vi "Find Midpoint.vi"(8 "error in (no error)":errorcluster, 10 "Image In":T1, 11 "Gantry Class in":refnum<class "Gantry Class.lvclass">) -> (0 "error out":errorcluster, 1 "Vec3d Class out":refnum<class "Vec3d Class.lvclass">, 2 "Image Out":T1, 3 "Gantry Class out":refnum<class "Gantry Class.lvclass">)   [LabVIEW 2017, in "Gantry Class.lvclass"]
uses:
  Gantry Class.lvclass
  Vec3d Class/Vec3d Class.lvclass
  Config Manager Class/Type Definitions/Camera Enum.ctl
  <vilib>/vision/Image Controls.llb/IMAQ Image.ctl
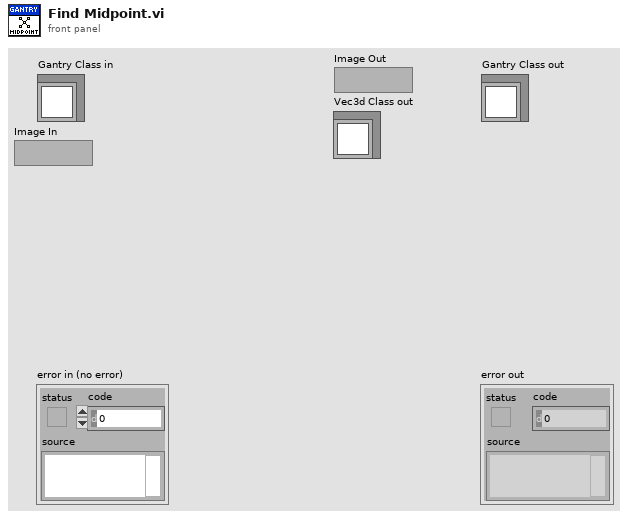
[diagram p1: front panel]
types:
  T1 = typedef "IMAQ Image.ctl" = refnum<image>
  T2 = typedef "Camera Enum.ctl" = enum16{"gantryhead", "NEEDLE CALIBRATION X", "NEEDLE CALIBRATION Y", "STAND CAMERA", "SIMRAN WEBCAM"}
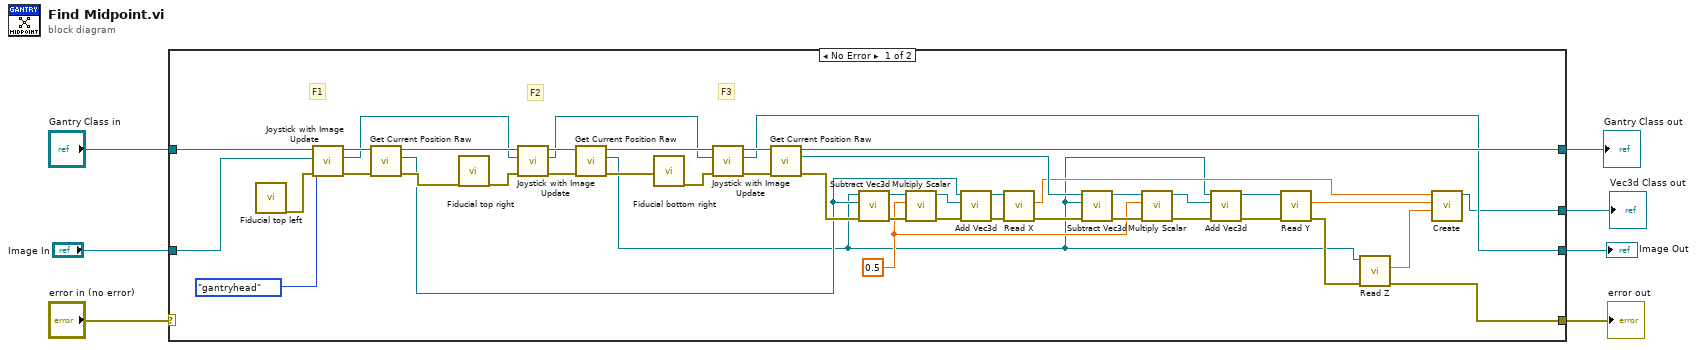
[diagram p0: block diagram]
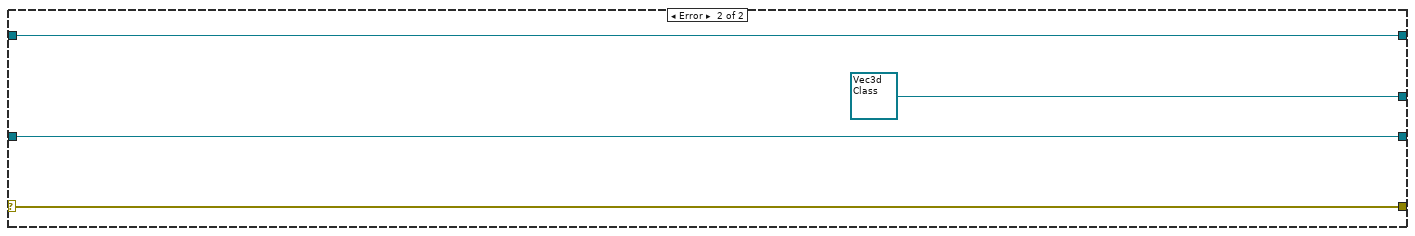
[diagram p2: hidden frame]
diagram:
  n1 = case shown="No Error" "error in (no error)" {
    selector: "error in (no error)" -> [_ w55]
    tunnel: [w24 w55] -> w6
    tunnel: "Gantry Class in" -> [w30 w54]
    tunnel: "Image In" -> [w29 w53]
    tunnel: [w26 w53] -> w3
    tunnel: [w27 w54] -> w2
    tunnel: [w20 refnum<class "Vec3d Class.lvclass"> refnum ("Vec3d Class out")] -> w1
    frame No Error {
      w12 = 0.5 ("Scale")
      # "F3"
      # "F2"
      # "F1"
      n2 = call "Fiducial top left"() -> ("error out"=w49:errorcluster)  [unwired: 18 in, 1 out]
      n3 = call-dynamic "Joystick with Image Update.vi"("error in (no error)"=w49, "Camera Name"=Camera_Enum."gantryhead", "Image In"=w29, "Gantry Class in"=w30) -> ("error out"=w50:errorcluster, "Image Out"=w32:T1, "Gantry Class out"=w51:refnum<class "Gantry Class.lvclass">)  [unwired: 5 in]
      n4 = call-dynamic "Get Current Position Raw.vi"("error in"=w50, "Gantry in"=w51) -> ("error out"=w44:errorcluster, "Vec3d Class out"=w10:refnum<class "Vec3d Class.lvclass">, "Gantry out"=w45:refnum<class "Gantry Class.lvclass">)  [unwired: 7 in]
      n5 = call "Fiducial top right"("error in (no error)"=w44) -> ("error out"=w46:errorcluster)  [unwired: 17 in, 1 out]
      n6 = call-dynamic "Joystick with Image Update.vi"("error in (no error)"=w46, "Image In"=w32, "Gantry Class in"=w45) -> ("error out"=w47:errorcluster, "Image Out"=w31:T1, "Gantry Class out"=w48:refnum<class "Gantry Class.lvclass">)  [unwired: 6 in]
      n7 = call-dynamic "Get Current Position Raw.vi"("error in"=w47, "Gantry in"=w48) -> ("error out"=w40:errorcluster, "Vec3d Class out"=w8:refnum<class "Vec3d Class.lvclass">, "Gantry out"=w39:refnum<class "Gantry Class.lvclass">)  [unwired: 7 in]
      n8 = call "Fiducial bottom right"("error in (no error)"=w40) -> ("error out"=w41:errorcluster)  [unwired: 17 in, 1 out]
      n9 = call-dynamic "Joystick with Image Update.vi"("error in (no error)"=w41, "Image In"=w31, "Gantry Class in"=w39) -> ("error out"=w42:errorcluster, "Image Out"=w26:T1, "Gantry Class out"=w43:refnum<class "Gantry Class.lvclass">)  [unwired: 6 in]
      n10 = call-dynamic "Get Current Position Raw.vi"("error in"=w42, "Gantry in"=w43) -> ("error out"=w34:errorcluster, "Vec3d Class out"=w37:refnum<class "Vec3d Class.lvclass">, "Gantry out"=w27:refnum<class "Gantry Class.lvclass">)  [unwired: 7 in]
      n11 = call "Subtract Vec3d.vi"("error in (no error)"=w34, "Vec3d in 2"=w10, "Vec3d in 1"=w8) -> ("error out"=w36:errorcluster, "Vec3d Class out"=w19:refnum<class "Vec3d Class.lvclass">)  [unwired: 7 in]
      n12 = call-dynamic "Multiply Scalar.vi"("error in"=w36, "Scale"=w12, "Vec3d in"=w19) -> ("error out"=w18:errorcluster, "Vec3d out"=w11:refnum<class "Vec3d Class.lvclass">)  [unwired: 7 in]
      n13 = call-dynamic "Add Vec3d.vi"("error in (no error)"=w18, 10:"Vec3d Class in"=w11, 11:"Vec3d Class in"=w10) -> ("error out"=w17:errorcluster, "Vec3d Class out"=w16:refnum<class "Vec3d Class.lvclass">)  [unwired: 7 in]
      n14 = call-dynamic "Read X.vi"("error in (no error)"=w17, "Vec3d Class in"=w16) -> ("error out"=w33:errorcluster, "X"=w23:dbl)  [unwired: 7 in, 1 out]
      n15 = call "Subtract Vec3d.vi"("error in (no error)"=w33, "Vec3d in 2"=w8, "Vec3d in 1"=w37) -> ("error out"=w35:errorcluster, "Vec3d Class out"=w38:refnum<class "Vec3d Class.lvclass">)  [unwired: 7 in]
      n16 = call-dynamic "Multiply Scalar.vi"("error in"=w35, "Scale"=w12, "Vec3d in"=w38) -> ("error out"=w15:errorcluster, "Vec3d out"=w9:refnum<class "Vec3d Class.lvclass">)  [unwired: 7 in]
      n17 = call-dynamic "Add Vec3d.vi"("error in (no error)"=w15, 10:"Vec3d Class in"=w9, 11:"Vec3d Class in"=w8) -> ("error out"=w13:errorcluster, "Vec3d Class out"=w14:refnum<class "Vec3d Class.lvclass">)  [unwired: 7 in]
      n18 = call-dynamic "Read Y.vi"("error in (no error)"=w13, "Vec3d Class in"=w14) -> ("error out"=w25:errorcluster, "Y"=w22:dbl)  [unwired: 7 in, 1 out]
      n19 = call-dynamic "Read Z.vi"("error in (no error)"=w25, "Vec3d Class in"=w8) -> ("error out"=w24:errorcluster, "Z"=w21:dbl)  [unwired: 7 in, 1 out]
      n20 = call "Create.vi"("Z"=w21, "Y"=w22, "X"=w23) -> ("Vec3d Class out"=w20:refnum<class "Vec3d Class.lvclass">)  [unwired: 7 in, 1 out]
    }
    frame Error {
    }
  }
  "error out" <- w6
  "Gantry Class out" <- w2
  "Image Out" <- w3
  "Vec3d Class out" <- w1
